vi "Create HTML Files.vi"(8 "error in (no error)":errorcluster, 10 "Topics":string[](array[string]), 11 "path":path) -> (0 "error out":errorcluster)   [LabVIEW 2015]
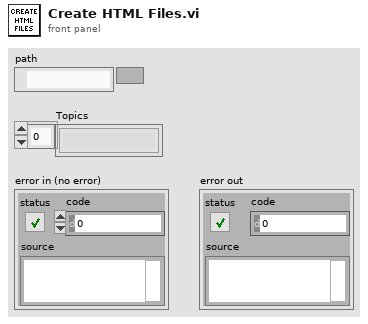
[diagram p1: front panel]
types:
  T1 = enum16{"open", "replace", "create", "open or create", "replace or create", "replace or create with confirmation"}
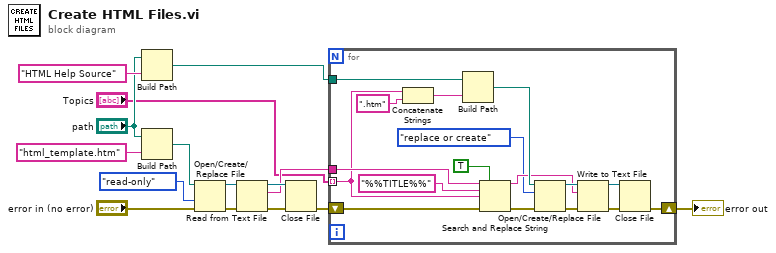
[diagram p0: block diagram]
diagram:
  n1 = Build Path(base path="path", name or relative path="HTML Help Source") -> (appended path=w5:path)
  n2 = Build Path(base path="path", name or relative path="html_template.htm" ("section")) -> (appended path=w7:path)
  n3 = Open/Create/Replace File(file path (use dialog)=w7, error in="error in (no error)", access (0:read/write)=enum16{"read/write", "read-only", "write-only"}."read-only") -> (refnum out=w9:refnum<file>, error out=w8:errorcluster)  [unwired: 3 in, 1 out]
  n4 = Read from Text File(file (use dialog)=w9, error in=w8) -> (refnum out=w12:refnum<file>, text=w10:string, error out=w11:errorcluster)  [unwired: 2 in, 1 out]
  n5 = Close File(refnum=w12, error in=w11) -> (error out=w14:errorcluster)  [unwired: 1 out]
  n6 = for {
    tunnel: "Topics" -> [w18] mode=indexing
    tunnel: w5 -> [w32]
    tunnel: w10 -> [w31]
    shift-right: [w20] -> w15
    shift-left: w14 -> [w22]
    n7 = Concatenate Strings(w18, ".htm" ("string")) -> (w16:string)
    n8 = Build Path(base path=w32, name or relative path=w16) -> (appended path=w28:path)
    n9 = Search and Replace String(replace all?=TRUE ("replace all? (F)"), input string=w31, search string="%%TITLE%%", replace string=w18, error in=w22) -> (result string=w23:string, error out=w21:errorcluster)  [unwired: 3 in, 2 out]
    n10 = Open/Create/Replace File(file path (use dialog)=w28, error in=w21, operation (0:open)=T1."replace or create") -> (refnum out=w26:refnum<file>, error out=w27:errorcluster)  [unwired: 3 in, 1 out]
    n11 = Write to Text File(file (use dialog)=w26, text=w23, error in=w27) -> (refnum out=w24:refnum<file>, error out=w25:errorcluster)  [unwired: 1 in, 1 out]
    n12 = Close File(refnum=w24, error in=w25) -> (error out=w20:errorcluster)  [unwired: 1 out]
  }
  "error out" <- w15
